vi "GetGroupsWithDynamicChannels.vi"(8 "error in (no error)":errorcluster, 10 "channels":T9[](array[typedef]), 11 "device configuration":T1) -> (0 "error out":errorcluster, 3 "groups with dynamic channels":string[](array[string]))   [LabVIEW 2017, in "CmsAcquisition.lvlib"]
uses:
  <vilib>/addons/InsightCM/Devices/Shared/Cms/CmsAcquisition/CmsAcquisition.lvlib
  <vilib>/addons/InsightCM/MessageBus/Base/controls/R2_Channel.ctl
  <vilib>/addons/InsightCM/MessageBus/Base/controls/KeyValuePair.ctl
  <vilib>/addons/InsightCM/MessageBus/Base/controls/Metric.ctl
  <vilib>/addons/InsightCM/MessageBus/Base/controls/R2_Device.ctl
  <vilib>/addons/InsightCM/MessageBus/Base/controls/DeviceState.ctl
  <vilib>/addons/InsightCM/MessageBus/Base/controls/R2_DataGroup.ctl
  <vilib>/addons/InsightCM/MessageBus/Base/controls/OperatingState.ctl
  <vilib>/addons/InsightCM/MessageBus/Base/controls/Trigger.ctl
  <vilib>/addons/InsightCM/MessageBus/Base/controls/Condition.ctl
  <vilib>/addons/InsightCM/MessageBus/Base/controls/BurstModeTrigger.ctl
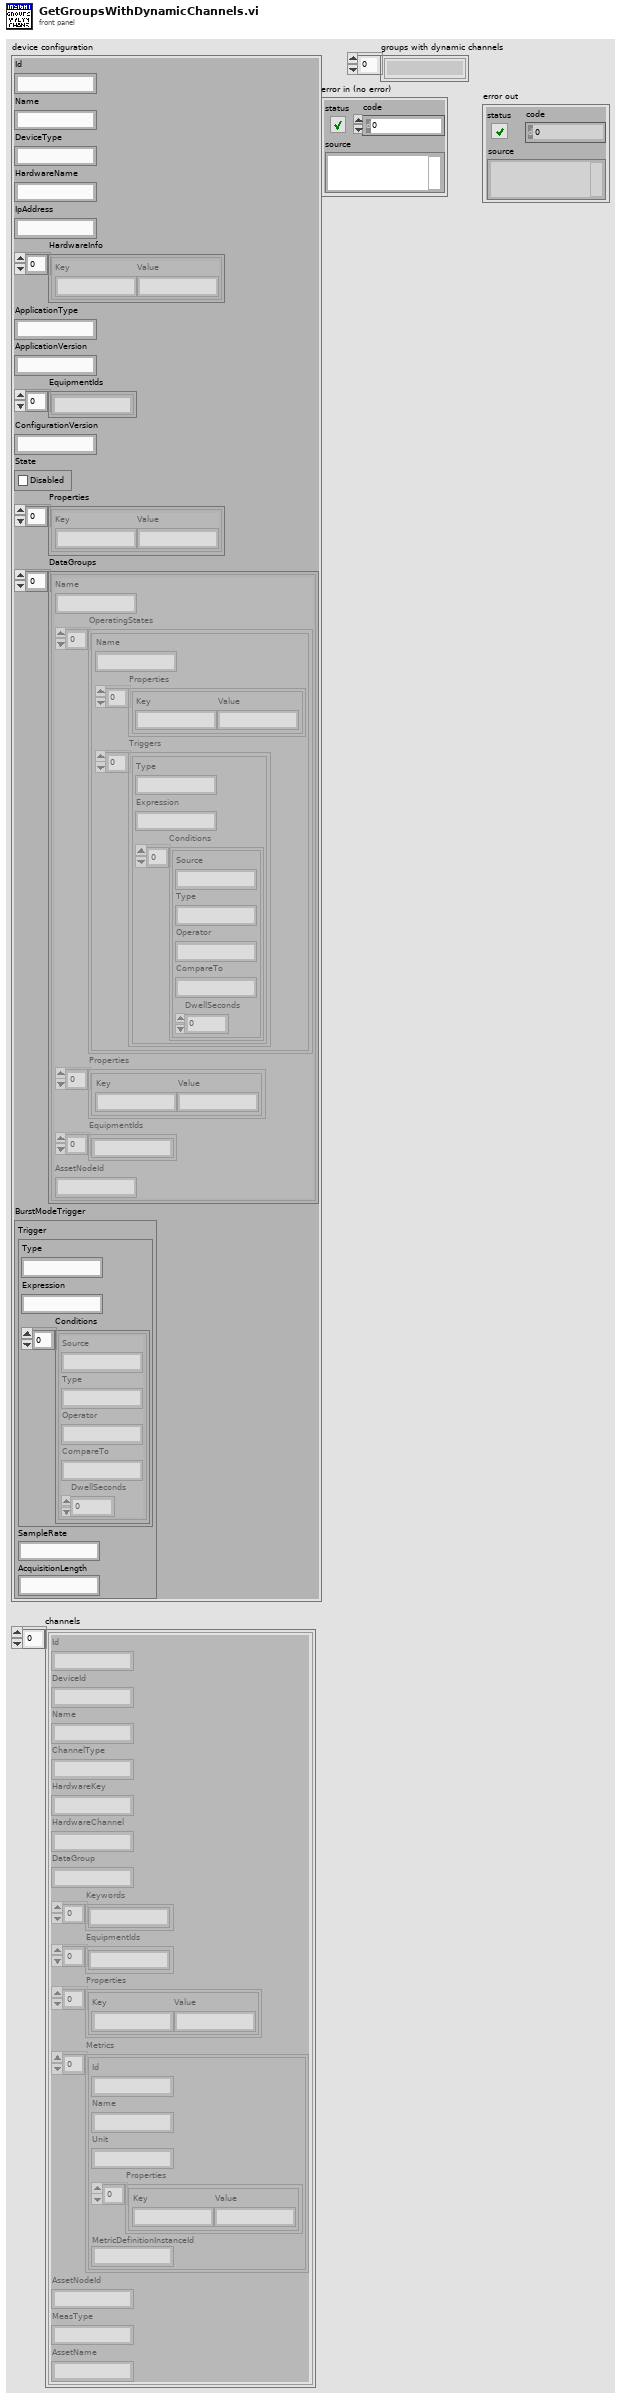
[diagram p1: front panel]
types:
  T1 = typedef "R2_Device.ctl" = cluster{"Id":string, "Name":string, "DeviceType":string, "HardwareName":string, "IpAddress":string, "HardwareInfo":T2[], "ApplicationType":string, "ApplicationVersion":string, "EquipmentIds":string[], "ConfigurationVersion":string, "State":T3, "Properties":T2[], "DataGroups":T4[], "BurstModeTrigger":T8}
  T2 = typedef "KeyValuePair.ctl" = cluster{"Key":string, "Value":string}
  T3 = typedef "DeviceState.ctl" = cluster{"Disabled":bool}
  T4 = typedef "R2_DataGroup.ctl" = cluster{"Name":string, "OperatingStates":T5[], "Properties":T2[], "EquipmentIds":string[], "AssetNodeId":string}
  T5 = typedef "OperatingState.ctl" = cluster{"Name":string, "Properties":T2[], "Triggers":T6[]}
  T6 = typedef "Trigger.ctl" = cluster{"Type":string, "Expression":string, "Conditions":T7[]}
  T7 = typedef "Condition.ctl" = cluster{"Source":string, "Type":string, "Operator":string, "CompareTo":string, "DwellSeconds":dbl}
  T8 = typedef "BurstModeTrigger.ctl" = cluster{"Trigger":T6, "SampleRate":string, "AcquisitionLength":string}
  T9 = typedef "R2_Channel.ctl" = cluster{"Id":string, "DeviceId":string, "Name":string, "ChannelType":string, "HardwareKey":string, "HardwareChannel":string, "DataGroup":string, "Keywords":string[], "EquipmentIds":string[], "Properties":T2[], "Metrics":T10[], "AssetNodeId":string, "MeasType":string, "AssetName":string}
  T10 = typedef "Metric.ctl" = cluster{"Id":string, "Name":string, "Unit":string, "Properties":T2[], "MetricDefinitionInstanceId":string}
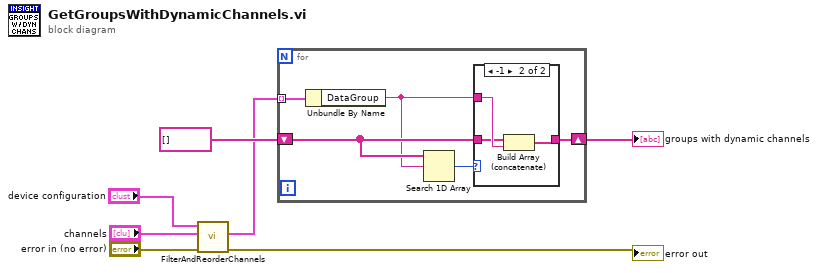
[diagram p0: block diagram]
diagram:
  n1 = call <vilib>:"FilterAndReorderChannels.vi"("error in (no error)"="error in (no error)", "channels"="channels", "device"="device configuration") -> ("error out"=→"error out":errorcluster, "acquisition channels (in acquisition order)"=w5:T9[])  [unwired: 7 in]
  n2 = for {
    tunnel: w5 -> [w12] mode=indexing
    shift-right: [w10] -> w6
    shift-left: string[] [] -> [w9]
    n3 = Unbundle By Name(w12) -> ("DataGroup"=w8:string)
    n4 = Search 1D Array(1D array=w9, element=w8) -> (index of element=w11:i32)  [unwired: 1 in]
    n5 = case shown="-1" w11 {
      tunnel: [w13 w14] -> w10
      tunnel: w9 -> [w13 w15]
      tunnel: w8 -> [_ w16]
      frame Default {
      }
      frame -1 {
        n6 = Build Array (concatenate)(w15, w16) -> (w14:string[])
      }
    }
  }
  "groups with dynamic channels" <- w6
